vi "ExecuteProgram.vi"(8 "error in (no error)":errorcluster, 9 "task id":i32(ring)=1 items=["TLibrary", "T01", "T02", "T03", "T04", "TAuxiliary"], 10 "path":path, 11 "controller in":refnum<k24>) -> (0 "error out":errorcluster, 2 "success":bool, 3 "controller out":refnum<k24>)   [LabVIEW 2016]
uses:
  C:/Program Files (x86)/Aerotech/Ensemble/LabVIEW/8.2/Bin/Aerotech.Ensemble.dll
  Bin/Aerotech.Ensemble.dll
  C:/Program Files (x86)/Aerotech/Ensemble/LabVIEW/8.2/Bin/Aerotech.Ensemble.LabVIEW.dll
  Bin/Aerotech.Ensemble.LabVIEW.dll
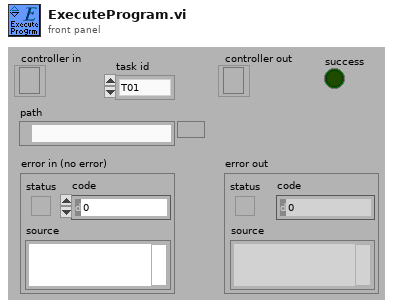
[diagram p1: front panel]
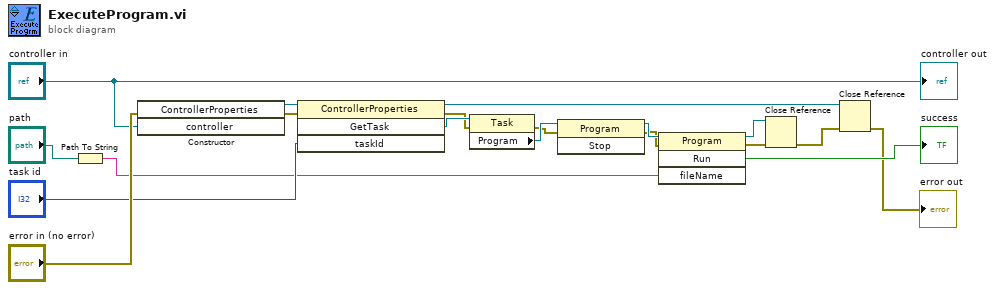
[diagram p0: block diagram]
diagram:
  n1 = Path To String(path="path") -> (string=w12:string)
  n2 = constructor class="ControllerProperties"(error in="error in (no error)", "controller"="controller in") -> (reference out=w16:refnum<k24>, error out=w15:errorcluster)  [unwired: 2 in, 2 out]
  n3 = invoke class="ControllerProperties" method="GetTask"(reference=w16, error in=w15, "taskId"="task id") -> (reference out=w14:refnum<k24>, error out=w5:errorcluster, "GetTask"=w6:refnum<k24>)  [unwired: 1 in, 1 out]
  n4 = property class="Task"(reference=w6, error in=w5) -> (error out=w2:errorcluster, "Program"=w4:refnum<k24>)  [unwired: 1 out]
  n5 = invoke class="Program" method="Stop"(reference=w4, error in=w2) -> (reference out=w3:refnum<k24>, error out=w1:errorcluster)  [unwired: 1 in, 1 out]
  n6 = invoke class="Program" method="Run"(reference=w3, error in=w1, "fileName"=w12) -> (reference out=w7:refnum<k24>, error out=w9:errorcluster, "Run"=→"success":bool)  [unwired: 1 in, 1 out]
  n7 = Close Reference(reference=w7, error in (no error)=w9) -> (error out=w8:errorcluster)
  n8 = Close Reference(reference=w14, error in (no error)=w8) -> (error out=→"error out":errorcluster)
  "controller out" <- "controller in"
